vi "Get Address.vi"(8 "Error in":errorcluster, 11 "10 - Bit Addressing in":refnum<class "10 - Bit Addressing.lvclass">) -> (0 "Error out":errorcluster, 3 "10 - Bit Addressing out":refnum<class "10 - Bit Addressing.lvclass">)   [LabVIEW 2020, in "10 - Bit Addressing.lvclass"]
uses:
  10 - Bit Addressing.lvclass
  C:/LV Assignments/SDLC VI/Class/Parent Class/Address/Address.lvclass
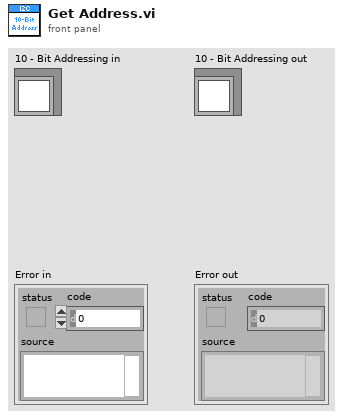
[diagram p1: front panel]
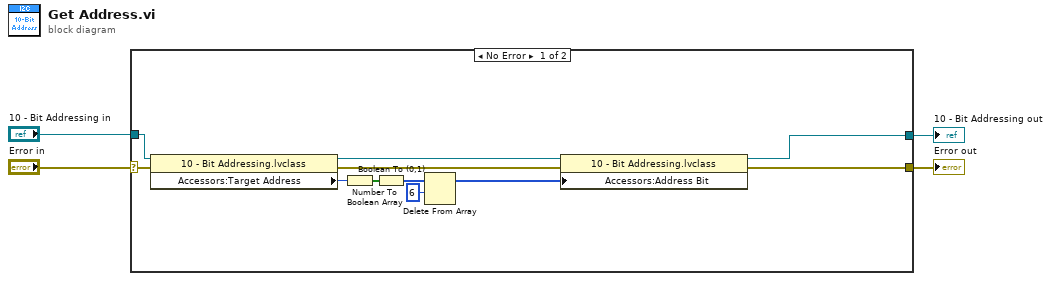
[diagram p0: block diagram]
diagram:
  n1 = case shown="No Error" "Error in" {
    selector: "Error in" -> [w15 w17]
    tunnel: [w10 w17] -> w3
    tunnel: [w5 w16] -> w1
    tunnel: "10 - Bit Addressing in" -> [w13 w16]
    frame No Error {
      n2 = property class="10 - Bit Addressing.lvclass"(reference=w13, error in=w15) -> (reference out=w9:refnum<class "10 - Bit Addressing.lvclass">, error out=w14:errorcluster, "Accessors:Target Address"=w12:i16)
      n3 = Number To Boolean Array(number=w12) -> (Boolean array=w11:bool[])
      n4 = Boolean To (0,1)(Boolean=w11) -> (0, 1=w8:i16[])
      n5 = Delete From Array(array=w8, length=6) -> (array with subset deleted=w6:i16[])  [unwired: 1 in, 1 out]
      n6 = property class="10 - Bit Addressing.lvclass"(reference=w9, error in=w14, "Accessors:Address Bit"=w6) -> (reference out=w5:refnum<class "10 - Bit Addressing.lvclass">, error out=w10:errorcluster)
    }
    frame Error {
    }
  }
  "Error out" <- w3
  "10 - Bit Addressing out" <- w1
